vi "Test ISO8601 Decimal Strings.vi"(8 "error in (no error)":errorcluster) -> (0 "error out":errorcluster)   [LabVIEW 2013]
uses:
  <vilib>/addons/_JKI Toolkits/Caraya/classes/Assert/Assert True.vi
  <vilib>/addons/_JKI Toolkits/Caraya/classes/Assert/Assert.lvclass
  <vilib>/addons/_JKI Toolkits/Caraya/classes/Test/Test.lvclass
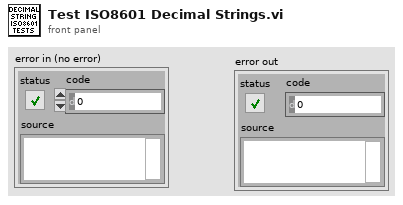
[diagram p1: front panel]
types:
  T1 = typedef "LVDateTimeRec.ctl" = cluster{"fractional second":dbl, "second":i32, "minute":i32, "hour":i32, "day of month":i32, "month":i32, "year":i32, "day of week":i32, "day of year":i32, "DST":i32}
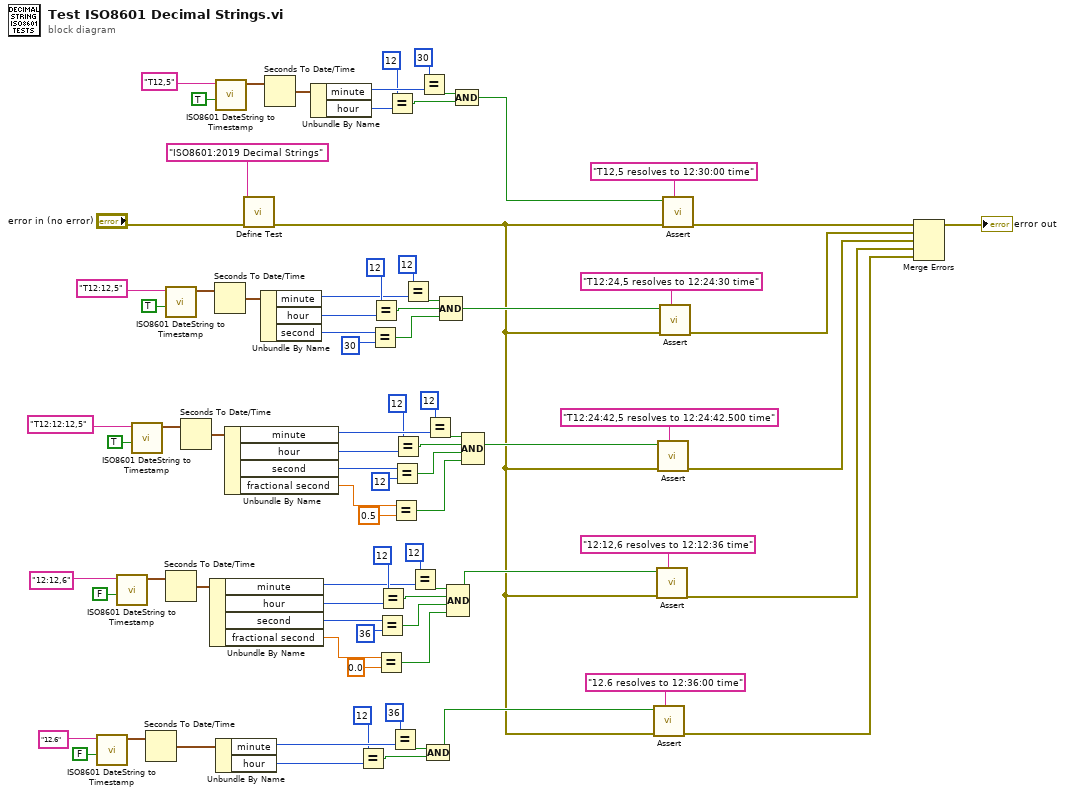
[diagram p0: block diagram]
diagram:
  n1 = call "ISO8601 DateString to Timestamp.vi"("Strict ISO? (T)"=FALSE, "ISO8601 Date String"="12.6" ("Label (VI Title)")) -> ("Timestamp"=w13:timestamp)  [unwired: 7 in, 2 out]
  n2 = call "ISO8601 DateString to Timestamp.vi"("Strict ISO? (T)"=FALSE, "ISO8601 Date String"="12:12,6" ("Label (VI Title)")) -> ("Timestamp"=w22:timestamp)  [unwired: 7 in, 2 out]
  n3 = call "ISO8601 DateString to Timestamp.vi"("Strict ISO? (T)"=TRUE, "ISO8601 Date String"="T12:12:12,5" ("Label (VI Title)")) -> ("Timestamp"=w49:timestamp)  [unwired: 7 in, 2 out]
  n4 = Seconds To Date/Time(time stamp (now)=w13) -> (date time rec=w12:T1)  [unwired: 1 in]
  n5 = call "ISO8601 DateString to Timestamp.vi"("Strict ISO? (T)"=TRUE, "ISO8601 Date String"="T12:12,5" ("Label (VI Title)")) -> ("Timestamp"=w63:timestamp)  [unwired: 7 in, 2 out]
  n6 = Seconds To Date/Time(time stamp (now)=w22) -> (date time rec=w23:T1)  [unwired: 1 in]
  n7 = Seconds To Date/Time(time stamp (now)=w49) -> (date time rec=w48:T1)  [unwired: 1 in]
  n8 = Unbundle By Name(w23) -> ("minute"=w24:i32, "hour"=w27:i32, "second"=w20:i32, "fractional second"=w31:dbl)
  n9 = Seconds To Date/Time(time stamp (now)=w63) -> (date time rec=w64:T1)  [unwired: 1 in]
  n10 = call "ISO8601 DateString to Timestamp.vi"("Strict ISO? (T)"=TRUE, "ISO8601 Date String"="T12,5" ("Label (VI Title)")) -> ("Timestamp"=w79:timestamp)  [unwired: 7 in, 2 out]
  n11 = Unbundle By Name(w12) -> ("minute"=w11:i32, "hour"=w8:i32)
  n12 = Unbundle By Name(w48) -> ("minute"=w47:i32, "hour"=w44:i32, "second"=w52:i32, "fractional second"=w36:dbl)
  n13 = call <vilib>:"Define Test.vi"("error in (no error)"="error in (no error)", "Label (VI Title)"="ISO8601:2019 Decimal Strings") -> ("error out"=w2:errorcluster)  [unwired: 8 in, 1 out]
  n14 = Unbundle By Name(w64) -> ("minute"=w65:i32, "hour"=w68:i32, "second"=w60:i32)
  n15 = Seconds To Date/Time(time stamp (now)=w79) -> (date time rec=w78:T1)  [unwired: 1 in]
  n16 = Unbundle By Name(w78) -> ("minute"=w77:i32, "hour"=w74:i32)
  n17 = Equal?(x=12, y=w8) -> (x = y?=w7:bool)
  n18 = Equal?(x=w60, y=30 ("x")) -> (x = y?=w58:bool)
  n19 = Equal?(x=12, y=w68) -> (x = y?=w69:bool)
  n20 = Equal?(x=w31, y=0.0) -> (x = y?=w33:bool)
  n21 = Equal?(x=w20, y=36 ("x")) -> (x = y?=w19:bool)
  n22 = Equal?(x=12, y=w27) -> (x = y?=w28:bool)
  n23 = Equal?(x=12, y=w74) -> (x = y?=w73:bool)
  n24 = Equal?(x=36, y=w11) -> (x = y?=w6:bool)
  n25 = Equal?(x=w36, y=0.5) -> (x = y?=w34:bool)
  n26 = Equal?(x=w52, y=12 ("x")) -> (x = y?=w53:bool)
  n27 = Equal?(x=12, y=w44) -> (x = y?=w43:bool)
  n28 = Equal?(x=12, y=w65) -> (x = y?=w70:bool)
  n29 = Equal?(x=12, y=w24) -> (x = y?=w29:bool)
  n30 = Equal?(x=30, y=w77) -> (x = y?=w72:bool)
  n31 = Equal?(x=12, y=w47) -> (x = y?=w42:bool)
  n32 = Compound Arithmetic op=AND(w6, w7) -> (w3:bool)
  n33 = Compound Arithmetic op=AND(w70, w69, w58) -> (w56:bool)
  n34 = Compound Arithmetic op=AND(w29, w28, w19, w33) -> (w16:bool)
  n35 = Compound Arithmetic op=AND(w72, w73) -> (w71:bool)
  n36 = Compound Arithmetic op=AND(w42, w43, w53, w34) -> (w55:bool)
  n37 = call-poly <vilib>:"Assert.vi"("Label"="12.6 resolves to 12:36:00 time" ("x"), "error in (no error)"=w2, "True?"=w3) -> ("error out"=w1:errorcluster)  [unwired: 7 in, 1 out]
  n38 = call-poly <vilib>:"Assert.vi"("Label"="12:12,6 resolves to 12:12:36 time" ("x"), "error in (no error)"=w2, "True?"=w16) -> ("error out"=w15:errorcluster)  [unwired: 7 in, 1 out]
  n39 = call-poly <vilib>:"Assert.vi"("Label"="T12:24:42,5 resolves to 12:24:42.500 time" ("x"), "error in (no error)"=w2, "True?"=w55) -> ("error out"=w39:errorcluster)  [unwired: 7 in, 1 out]
  n40 = call-poly <vilib>:"Assert.vi"("Label"="T12:24,5 resolves to 12:24:30 time" ("x"), "error in (no error)"=w2, "True?"=w56) -> ("error out"=w40:errorcluster)  [unwired: 7 in, 1 out]
  n41 = call-poly <vilib>:"Assert.vi"("Label"="T12,5 resolves to 12:30:00 time" ("x"), "error in (no error)"=w2, "True?"=w71) -> ("error out"=w41:errorcluster)  [unwired: 7 in, 1 out]
  n42 = Merge Errors(w41, w40, w39, w15, w1) -> (→"error out":errorcluster)
